vi "visaQuery.vi"(8 "error constant":errorcluster, 9 "disconnectPBot_Event":refnum<user-event>, 10 "stringToWrite":string, 11 "VISA resource name":refnum<visa-resource-name>) -> (0 "error Out":errorcluster, 2 "String":string, 3 "dub: VISA resource name":refnum<visa-resource-name>)   [LabVIEW 2015]
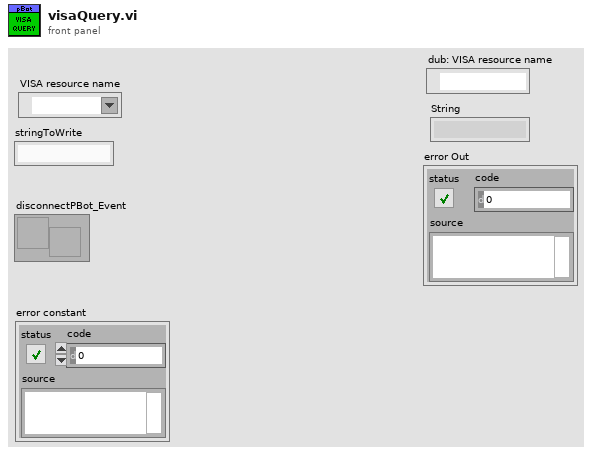
[diagram p1: front panel]
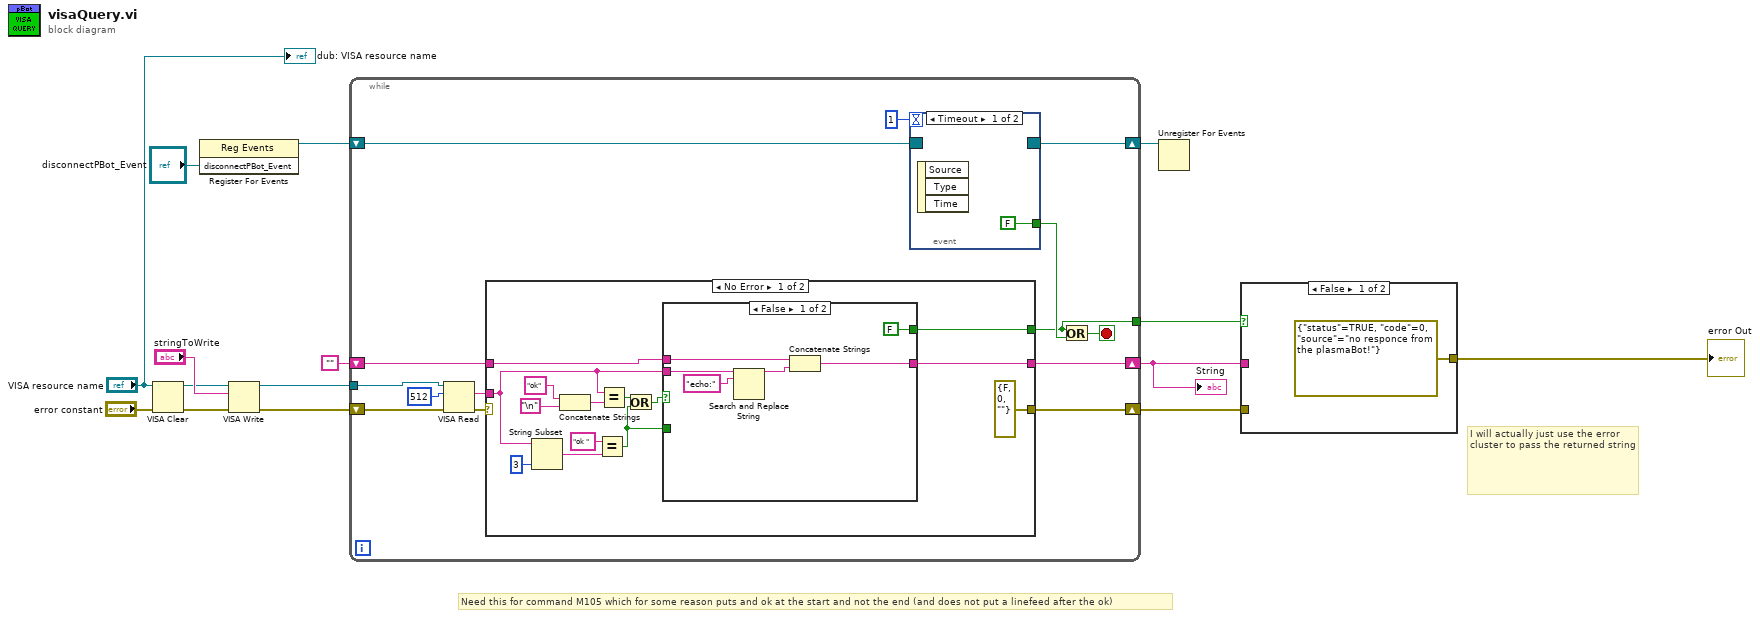
[diagram p0: block diagram]
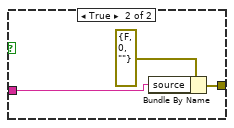
[diagram p2: hidden frame]
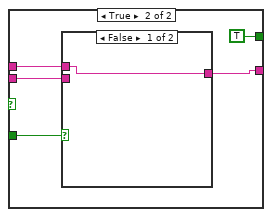
[diagram p3: hidden frame]
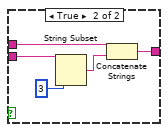
[diagram p4: hidden frame]
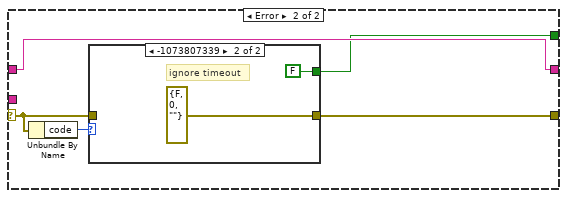
[diagram p5: hidden frame]
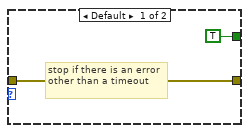
[diagram p6: hidden frame]
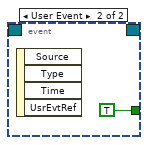
[diagram p7: hidden frame]
diagram:
  # "Need this for command M105 which for some reason puts and ok at the start and not the end (and does not put a linefeed after the ok)"
  # "I will actually just use the error cluster to pass the returned string"
  n1 = VISA Clear(VISA resource name="VISA resource name", error in (no error)="error constant") -> (VISA resource name out=w2:refnum<visa-resource-name>, error out=w3:errorcluster)
  n2 = register-events("disconnectPBot_Event") -> (reference out=w6:refnum<event-registration>)  [unwired: 2 in, 1 out]
  n3 = VISA Write(VISA resource name=w2, write buffer="stringToWrite", error in (no error)=w3) -> (VISA resource name out=w14:refnum<visa-resource-name>, error out=w13:errorcluster)  [unwired: 1 out]
  n4 = while {
    tunnel: w14 -> [w29]
    shift-right: [w16] -> w9
    shift-left: w13 -> [w28]
    shift-right: [w26] -> w8
    shift-left: "" -> [w27]
    tunnel: [w19] -> w11
    shift-right: [w21] -> w5
    shift-left: w6 -> [w22]
    stop <- w24 stop-if-true
    n5 = VISA Read(VISA resource name=w29, byte count=u32 512, error in (no error)=w28) -> (read buffer=w18:string, error out=w17:errorcluster)  [unwired: 2 out]
    n6 = case shown="No Error" w17 {
      selector: w17 -> [_ w63]
      tunnel: w27 -> [w43 w62]
      tunnel: [w42 w62] -> w26
      tunnel: [w41 w61] -> w19
      tunnel: w18 -> [w37 _]
      tunnel: [errorcluster {"status"=FALSE, "code"=0, "source"=""} ("error out") w64] -> w16
      frame No Error {
        n7 = String Subset(string=w37, length (rest)=3 ("length (rest)")) -> (substring=w34:string)  [unwired: 1 in]
        n8 = Concatenate Strings("ok" ("y"), "\n") -> (w39:string)
        n9 = Equal?(x="ok ", y=w34) -> (x = y?=w31:bool)
        n10 = Equal?(x=w37, y=w39) -> (x = y?=w32:bool)
        n11 = Or(x=w32, y=w31) -> (x .or. y?=w33:bool)
        n12 = case shown="False" w33 {
          tunnel: [FALSE TRUE] -> w41
          tunnel: w43 -> [w49 w52]
          tunnel: w37 -> [w46 w51]
          tunnel: [w48 w50] -> w42
          tunnel: w31 -> [_ w53]
          frame False {
            n13 = Search and Replace String(input string=w46, search string="echo:") -> (result string=w47:string)  [unwired: 6 in, 3 out]
            n14 = Concatenate Strings(w49, w47) -> (w48:string)
          }
          frame True {
            n15 = case shown="False" w53 {
              tunnel: w52 -> [w55 w60]
              tunnel: w51 -> [_ w58]
              tunnel: [w55 w59] -> w50
              frame False {
              }
              frame True {
                # "Most likely M105 was send which for some reason puts and ok at the start and not the end"
                n16 = String Subset(string=w58, offset (0)=3) -> (substring=w56:string)  [unwired: 1 in]
                n17 = Concatenate Strings(w60, w56) -> (w59:string)
              }
            }
          }
        }
      }
      frame Error {
        n18 = Unbundle By Name(w63) -> ("code"=w65:i32)
        n19 = case shown="-1073807339" w65 {
          tunnel: w63 -> [w67 _]
          tunnel: [w67 errorcluster {"status"=FALSE, "code"=0, "source"=""} ("error out")] -> w64
          tunnel: [TRUE FALSE] -> w61
          frame Default {
            # "stop if there is an error other than a timeout"
          }
          frame -1073807339 {
            # "ignore timeout"
          }
        }
      }
    }
    n20 = event shown="[0] Timeout" {
      selector: w22 -> [_ _]
      dyn-events: [_ _] -> w21
      timeout: 1 -> [_ _]
      tunnel: [FALSE TRUE] -> w20
      event Timeout {
        n21 = event-data() -> ()  [unwired: 1 in, 3 out]
      }
      event User Event {
        n22 = event-data() -> ()  [unwired: 1 in, 4 out]
      }
    }
    n23 = Or(x=w19, y=w20) -> (x .or. y?=w24:bool)
  }
  "String" <- w8
  n24 = Unregister For Events(event registration refnum=w5) -> ()  [unwired: 1 in, 1 out]
  n25 = case shown="False" w11 {
    tunnel: [errorcluster {"status"=TRUE, "code"=0, "source"="no responce from the plasmaBot!"} ("error constant") w73] -> w10
    tunnel: w9 -> [_ _]
    tunnel: w8 -> [_ w74]
    frame False {
    }
    frame True {
      n26 = Bundle By Name(cluster=errorcluster {"status"=FALSE, "code"=0, "source"=""} ("error constant"), "source"=w74) -> (w73:errorcluster)
    }
  }
  "error Out" <- w10
  "dub: VISA resource name" <- "VISA resource name"
